vi "PCSMain.Free PHELIX BB Instances.vi"(1 "DB Entries":cluster{"Object Name":string, "Class":string}[](array[cluster])) -> (0 "Free BB Instances":cluster{"Object Name":string, "Class":string}[](array[cluster]))   [LabVIEW 2014, in "PCSMain.lvlib"]
doc: "This VI acts as a filter: From the input data base entries, it gives out all which are belonging to the class PH_BlackBox except those named inside the block diagram. This VI is meant to be used in MainGUIs."
uses:
  PCSMain.lvlib
  PH_Beamline/PH_Beamline.Black Box Instances.ctl
  Z6_Beamline/Z6_Beamline.Black Box Instances.ctl
  PH_Beamline/PH_Beamline.lvlib
  Z6_Beamline/Z6_Beamline.lvlib
panel:
  in  "Z6 Black Box Instances":T1="Z6_ST_Attenuator_1_BB"
  in  "Black Box Instances":T2="PA_CH1_BB"
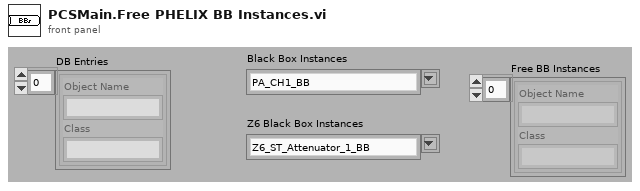
[diagram p1: front panel]
types:
  T1 = typedef "Z6_Beamline.lvlib/Z6_Beamline.Black Box Instances.ctl" = string
  T2 = typedef "PH_Beamline.lvlib/PH_Beamline.Black Box Instances.ctl" = string
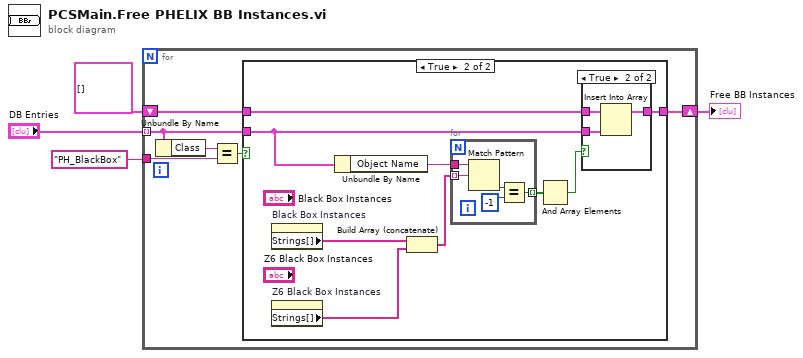
[diagram p0: block diagram]
diagram:
  n1 = for {
    tunnel: "PH_BlackBox" ("Class") -> [w10]
    tunnel: "DB Entries" -> [w8] mode=indexing
    shift-right: [w6] -> w4
    shift-left: cluster{"Object Name":string, "Class":string}[] [] -> [w5]
    n2 = Unbundle By Name(w8) -> ("Class"=w7:string)
    n3 = Equal?(x=w7, y=w10) -> (x = y?=w9:bool)
    n4 = case shown="True" w9 {
      tunnel: w8 -> [_ w16]
      tunnel: [w11 w20] -> w6
      tunnel: w5 -> [w11 w19]
      frame False {
      }
      frame True {
        n5 = property on="Black Box Instances" class="CmbBox (strict)"() -> ("Strings[]"=w13:string[])  [unwired: 2 in, 2 out]
        n6 = property on="Z6 Black Box Instances" class="CmbBox (strict)"() -> ("Strings[]"=w12:string[])  [unwired: 2 in, 2 out]
        n7 = Unbundle By Name(w16) -> ("Object Name"=w18:string)
        n8 = Build Array (concatenate)(w13, w12) -> (w14:string[])
        n9 = for {
          tunnel: w18 -> [w25]
          tunnel: w14 -> [w24] mode=indexing
          tunnel: [w21] -> w17 mode=indexing
          n10 = Match Pattern(string=w25, regular expression=w24) -> (offset past match=w23:i32)  [unwired: 1 in, 3 out]
          n11 = Equal?(x=w23, y=-1) -> (x = y?=w21:bool)
        }
        n12 = And Array Elements(Boolean array=w17) -> (logical AND=w15:bool)
        n13 = case shown="True" w15 {
          tunnel: w16 -> [_ w29]
          tunnel: [w26 w28] -> w20
          tunnel: w19 -> [w26 w27]
          frame False {
          }
          frame True {
            n14 = Insert Into Array(array=w27, new element=w29) -> (w28:cluster{"Object Name":string, "Class":string}[])  [unwired: 1 in]
          }
        }
      }
    }
  }
  "Free BB Instances" <- w4
